vi "Overall_system_A0-4_Weightfirst_w_LoadCell_1RFID.vi"() -> ()   [LabVIEW 2019]
doc: "This VI is th overall VI that can read the weight, rfid and camera (and save the data into a csv file). When certain threshold are met it can also send a telegram message at the end."
uses:
  dependencies/notification/Telegram-Bot-master (1)/Telegram-Bot-master/Telegram/Methods/TypeDefs/SendMessageType.ctl
panel:
  out "Rfid":string
  in  "RFID VISA resource name":refnum<visa-resource-name>="COM5"
  in  "start rfid (debug)":bool
  out "Triggered/Past Weight":string
  in  "Weight VISA resource name":refnum<visa-resource-name>="COM1"
  in  "start condition (debug)":bool
  in  "Start camera (debug)":bool
  out "Health Monitoring in Progress":bool
  in  "Bird is underfeeding (debug)":bool
  out "Current image":T1(plugin-control)
  in  "Camera Name":refnum<k21>="cam0" caption="IMAQdx Session"
  # "Intelligent Health Monitoring System"
  # "grams"
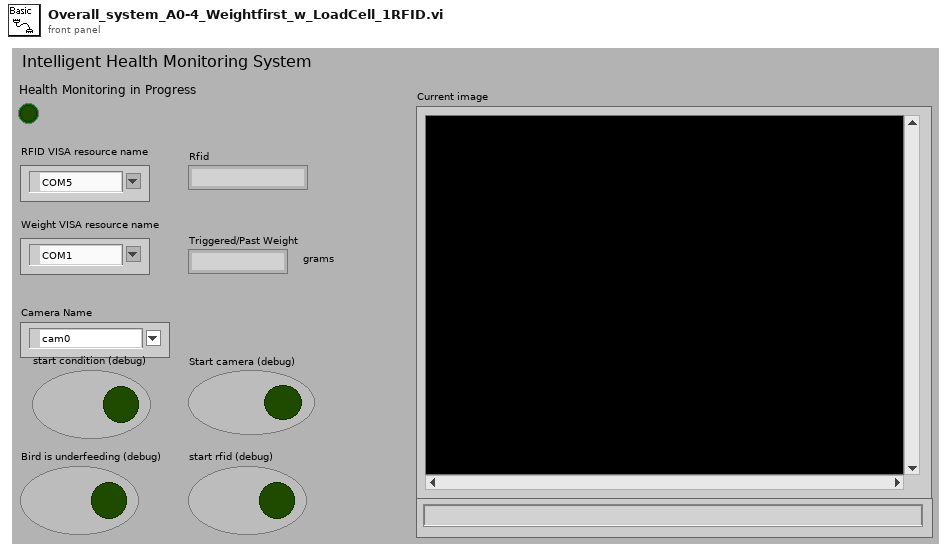
[diagram p1: front panel]
types:
  T1 = typedef "IMAQ Image.ctl" = refnum<image>
  T2 = typedef "SendMessageType.ctl" = enum16{"Text", "ReplyKeyboardMarkup", "ReplyKeyboardRemove"}
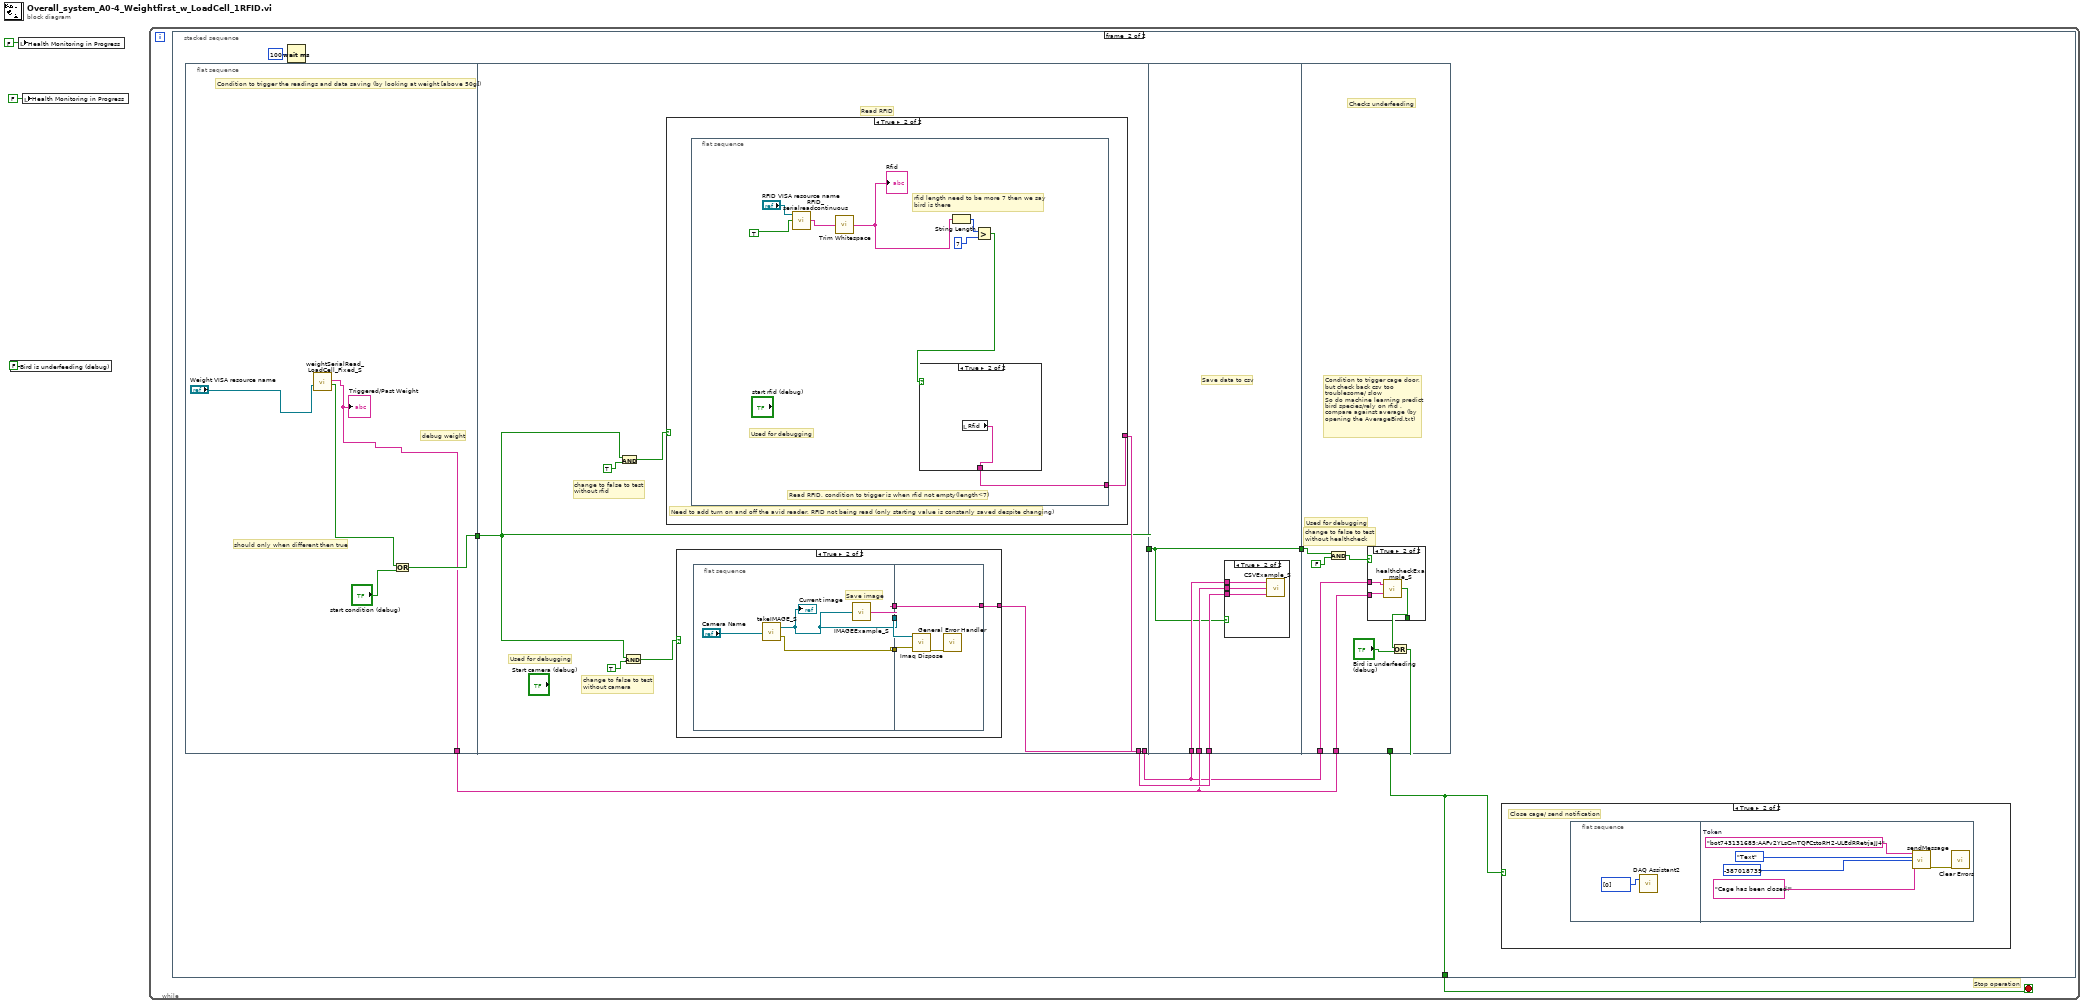
[diagram p0: block diagram]
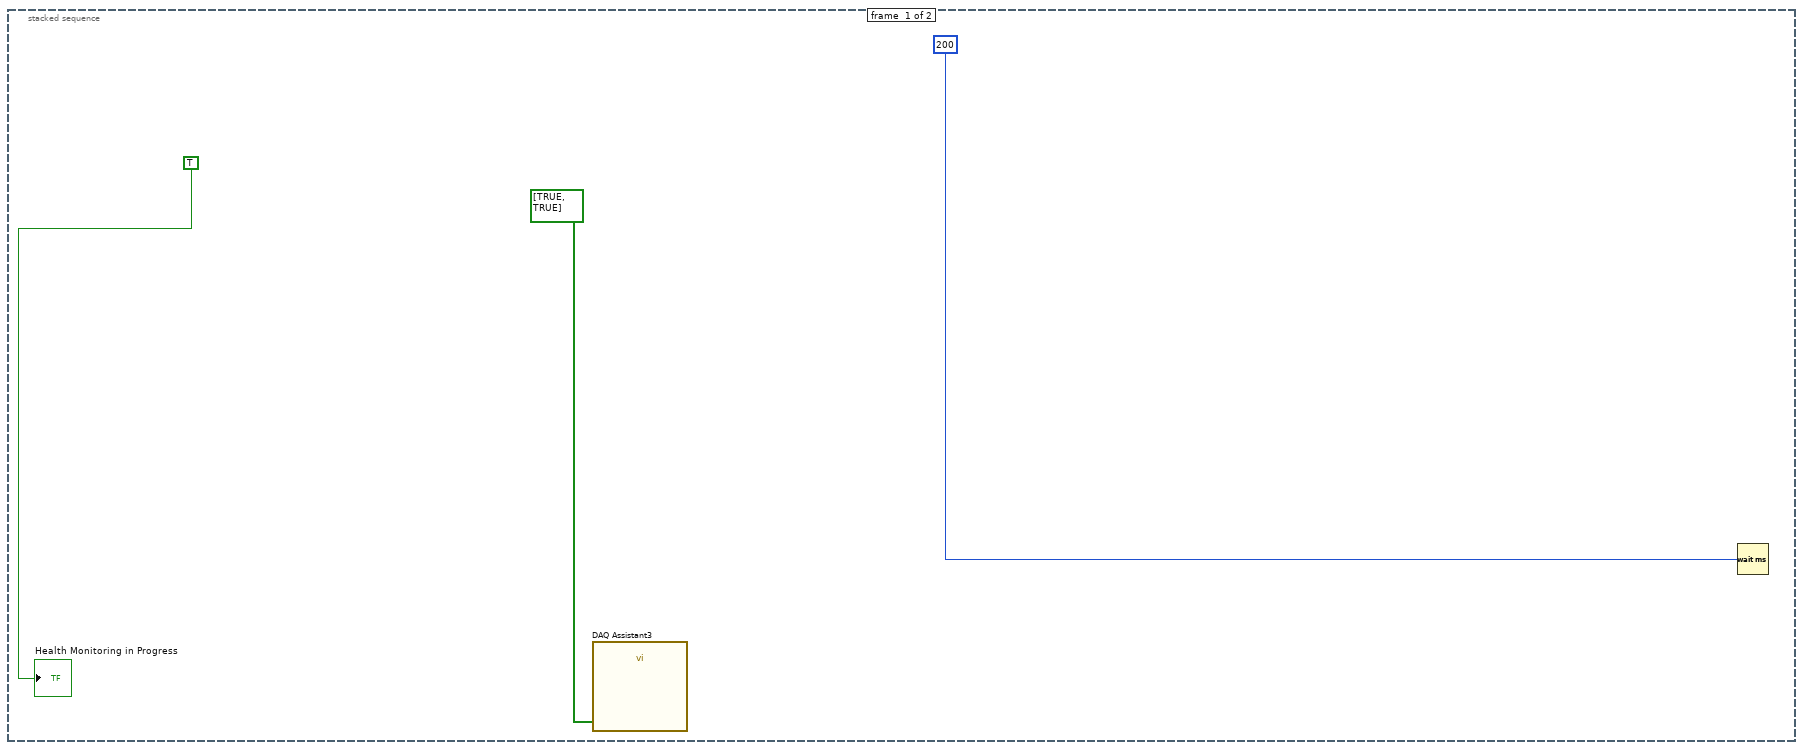
[diagram p2: hidden frame]
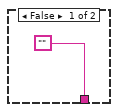
[diagram p5: hidden frame]
diagram:
  n1 = local write "Bird is underfeeding (debug)"(FALSE ("Bird is underfeeding")) -> ()
  n2 = local write "Health Monitoring in Progress"(FALSE ("Health Monitoring in Progress")) -> ()
  n3 = local write "Health Monitoring in Progress"(FALSE ("Health Monitoring in Progress")) -> ()
  n4 = while {
    stop <- w4 stop-if-true
    # "Stop operation"
    n5 = stacked-sequence {
      tunnel: [_ w14] -> w4
      frame #0 {
        n6 = call "DAQ Assistant3"("data"=bool[] [TRUE, TRUE]) -> ()  [unwired: 17 in, 2 out]
        n7 = Wait (ms)(milliseconds to wait=u32 200) -> ()  [unwired: 1 out]
        "Health Monitoring in Progress" <- TRUE ("Health Monitoring in Progress")
      }
      frame #1 {
        n8 = flat-sequence {
          tunnel: [w18] -> w9
          tunnel: [w19] -> w13
          tunnel: [w27] -> w8
          tunnel: [w26] -> w10
          tunnel: w13 -> [w22]
          tunnel: [w22] -> w12
          tunnel: w12 -> [w51]
          tunnel: [w51] -> w11
          tunnel: w10 -> [w54]
          tunnel: w9 -> [w53]
          tunnel: w8 -> [w52]
          tunnel: [w61] -> w14
          tunnel: w9 -> [w65]
          tunnel: w11 -> [w58]
          tunnel: w8 -> [w64]
          frame #0 {
            # "debug weight"
            # "Condition to trigger the readings and data saving (by looking at weight [above 50g])"
            # "should only when different then true"
            n9 = call "weightSerialRead_LoadCell_Fixed_S.vi"("VISA resource name"="Weight VISA resource name") -> ("Boolean"=w17:bool, "Current Weight"=w18:string)  [unwired: 9 in]
            "Triggered/Past Weight" <- w18
            n10 = Or(x=w17, y="start condition (debug)") -> (x .or. y?=w19:bool)
          }
          frame #1 {
            # "change to false to test \nwithout rfid"
            # "change to false to test \nwithout camera"
            # "Used for debugging"
            # "Read RFID"
            n11 = And(x=w22, y=TRUE) -> (x .and. y?=w21:bool)
            n12 = And(x=w22, y=TRUE) -> (x .and. y?=w24:bool)
            n13 = case shown="True" w21 {
              tunnel: [_ w40] -> w27
              frame False {
              }
              frame True {
                # "Need to add turn on and off the avid reader, RFID not being read (only starting value is constanly saved despite changing)"
                n14 = flat-sequence {
                  tunnel: [w42] -> w40
                  frame #0 {
                    # "Used for debugging"
                    # "rfid length need to be more 7 then we say \nbird is there"
                    # "Read RFID, condition to trigger is when rfid not empty(length<7)"
                    n15 = call "RFID_serialreadcontinuous.vi"("Read 2"=TRUE, "VISA resource name"="RFID VISA resource name") -> ("Response 2"=w45:string)  [unwired: 1 in]
                    n16 = call <vilib>:"Trim Whitespace.vi"("string"=w45) -> ("trimmed string"=w46:string)  [unwired: 1 in]
                    "Rfid" <- w46
                    n17 = String Length(string=w46) -> (length=w48:i32)
                    n18 = Greater?(x=w48, y=7) -> (0:w41:bool)
                    n19 = case shown="True" w41 {
                      tunnel: ["" w50] -> w42
                      frame False {
                      }
                      frame True {
                        n20 = local read "Rfid"() -> (w50:string)
                      }
                    }
                  }
                }
              }
            }
            n21 = case shown="True" w24 {
              tunnel: [_ w29] -> w26
              frame False {
              }
              frame True {
                n22 = flat-sequence {
                  tunnel: [w33] -> w31
                  tunnel: [w32] -> w30
                  tunnel: [w35] -> w28
                  tunnel: w31 -> [w39]
                  tunnel: w30 -> [w37]
                  tunnel: [w36] -> w29
                  tunnel: w28 -> [w36]
                  frame #0 {
                    # "Save image"
                    n23 = call "takeIMAGE_S.vi"("Camera Name"="Camera Name") -> ("Current image"=w32:T1, "error in (no error)"=w33:errorcluster)
                    "Current image" <- w32
                    n24 = call "IMAGEExample_S.vi"("Image"=w32) -> ("String"=w35:string)
                  }
                  frame #1 {
                    n25 = call "Imaq Dispose"("Image"=w37, "error in (no error)"=w39) -> ("error out"=w38:errorcluster)  [unwired: 4 in]
                    n26 = call <vilib>:"General Error Handler.vi"("error in (no error)"=w38) -> ()  [unwired: 2 in, 13 out]
                  }
                }
              }
            }
          }
          frame #2 {
            # "Save data to csv"
            n27 = case shown="True" w51 {
              tunnel: w54 -> [_ w55]
              tunnel: w53 -> [_ w56]
              tunnel: w52 -> [_ w57]
              frame False {
              }
              frame True {
                n28 = call "CSVExample_S.vi"("imageId"=w55, "weight"=w56, "rfid"=w57) -> ()
              }
            }
          }
          frame #3 {
            # "change to false to test \nwithout healthcheck"
            # "Used for debugging"
            # "Condition to trigger cage door,\nbut check back csv too troublesome/ slow\nSo do machine learning predict bird species/rely on rfid , compare against average (by opening the AverageBird.txt)"
            # "Checks underfeeding"
            n29 = And(x=w58, y=FALSE) -> (x .and. y?=w59:bool)
            n30 = case shown="True" w59 {
              tunnel: [_ w66] -> w63
              tunnel: w64 -> [_ w67]
              tunnel: w65 -> [_ w68]
              frame False {
              }
              frame True {
                n31 = call "healthcheckExample_S.vi"("weight"=w68, "rfid"=w67) -> ("Boolean"=w66:bool)
              }
            }
            n32 = Or(x=w63, y="Bird is underfeeding (debug)") -> (x .or. y?=w61:bool)
          }
        }
        n33 = Wait (ms)(milliseconds to wait=u32 100) -> ()  [unwired: 1 out]
        n34 = case shown="True" w14 {
          frame False {
          }
          frame True {
            # "Close cage/ send notification"
            n35 = flat-sequence {
              frame #0 {
                n36 = call "DAQ Assistant2"("data"=u32[] [0]) -> ()  [unwired: 17 in, 2 out]
              }
              frame #1 {
                w73 = "bot743131685:AAFv2YLsCmTQFCztoRH2-ULEdRRetrjaJJ4"  # Token
                n37 = call "sendMessage.vi"("Token"=w73, "MsgType"=SendMessageType."Text", "ChatId"=i64 -387018739, "Text"="Cage has been closed!") -> ("error out"=w74:errorcluster)  [unwired: 11 in]
                n38 = call <vilib>:"Clear Errors.vi"("error in (no error)"=w74) -> ()  [unwired: 5 in, 2 out]
              }
            }
          }
        }
      }
    }
  }
